vi "lock vis.vi"(10 "parameters":variant[](array[variant]), 11 "vis":refnum<vi>[](array[refnum])) -> (0 "error report":errorcluster[](array[cluster]))   [LabVIEW 2013]
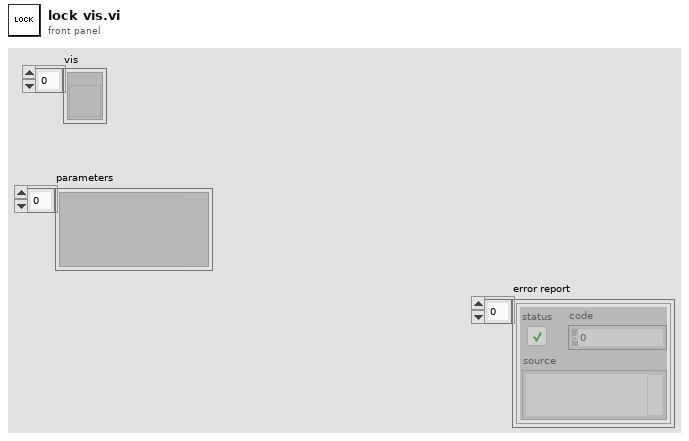
[diagram p1: front panel]
types:
  T1 = enum32{"invalid lock state", "Not Locked", "Locked (No Password)", "Password-protected"}
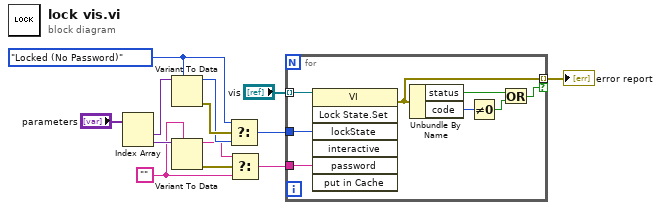
[diagram p0: block diagram]
diagram:
  w2 = ""
  w6 = T1."Locked (No Password)" ("Lock State")
  n1 = Index Array(array="parameters") -> (element #1=w10:variant, element #2=w4:variant)  [unwired: 2 in]
  n2 = Variant To Data(type=w6, Variant=w10) -> (data=w8:T1, error out=w9:errorcluster)  [unwired: 1 in]
  n3 = Variant To Data(type=w2, Variant=w4) -> (data=w3:string, error out=w5:errorcluster)  [unwired: 1 in]
  n4 = Select(t=w6, s=w9, f=w8) -> (s? t:f=w7:T1)
  n5 = Select(t=w3, s=w5, f=w2) -> (s? t:f=w1:string)
  n6 = for {
    tunnel: "vis" -> [w17] mode=indexing
    tunnel: [w16] -> w12 mode=indexing if=w18
    tunnel: w7 -> [w15]
    tunnel: w1 -> [w14]
    n7 = invoke class="VI" method="Lock State.Set"(reference=w17, "lockState"=w15, "password"=w14) -> (error out=w16:errorcluster)  [unwired: 4 in, 6 out]
    n8 = Unbundle By Name(w16) -> ("status"=w21:bool, "code"=w20:i32)
    n9 = Not Equal To 0?(x=w20) -> (x != 0?=w19:bool)
    n10 = Or(x=w21, y=w19) -> (x .or. y?=w18:bool)
  }
  "error report" <- w12
